vi "get_multiramp_soak_segment_event_configuration.vi"(8 "error in (no error)":errorcluster, 10 "Segment number":u8 max=15, 11 "VISA Refnum in":refnum<visa-resource-name>) -> (0 "error out":errorcluster, 1 "Soak enabled":bool, 2 "Ramp enabled":bool, 3 "VISA Refnum out":refnum<visa-resource-name>)   [LabVIEW 2018]
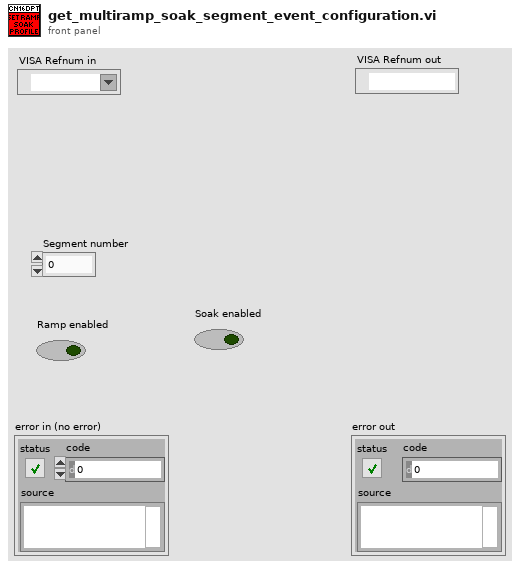
[diagram p1: front panel]
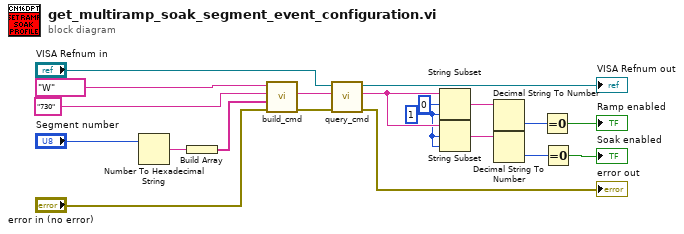
[diagram p0: block diagram]
diagram:
  w7 = 1 ("length (rest)")
  n1 = Number To Hexadecimal String(2:"Segment number") -> (0:w10:string)  [unwired: 1 in]
  n2 = Build Array(w10) -> (w12:string[])
  n3 = call "build_cmd.vi"("error in (no error)"="error in (no error)", "Parameter list"=w12, "Command ID"="730", "Command class"="W") -> ("error out"=w15:errorcluster, "Command"=w14:string)  [unwired: 6 in]
  n4 = call "query_cmd.vi"("error in (no error)"=w15, "Command"=w14, "VISA resource name"="VISA Refnum in") -> ("error out"=→"error out":errorcluster, "Response"=w9:string, "VISA resource name out"=→"VISA Refnum out":refnum<visa-resource-name>)  [unwired: 6 in]
  n5 = String Subset(string=w9, offset (0)=0, length (rest)=w7) -> (substring=w6:string)
  n6 = String Subset(string=w9, offset (0)=w7, length (rest)=w7) -> (substring=w5:string)
  n7 = Decimal String To Number(string=w6) -> (number=w4:i32)  [unwired: 2 in, 1 out]
  n8 = Decimal String To Number(string=w5) -> (number=w3:i32)  [unwired: 2 in, 1 out]
  n9 = Equal To 0?(x=w4) -> (x = 0?=→"Ramp enabled":bool)
  n10 = Equal To 0?(x=w3) -> (x = 0?=→"Soak enabled":bool)
